vi "VCS Get Velocity Regulator Feed Forward.vi"(0 "axis in":cluster{"keyHandle":u32, "nodeId":u16}={"keyHandle"=0, "nodeId"=1}, 11 "error in (no error)":errorcluster) -> (4 "axis out":cluster{"keyHandle":u32, "nodeId":u16}={"keyHandle"=0, "nodeId"=1}, 6 "feed forward":T1, 15 "error out":errorcluster)   [LabVIEW 2010]
doc: "<B>VCS_GetVelocityRegulatorFeedForward</B> reads parameters for velocity regulation feed forward."
uses:
  Resources/EposCmd.dll
  Resources/EposCmd64.dll
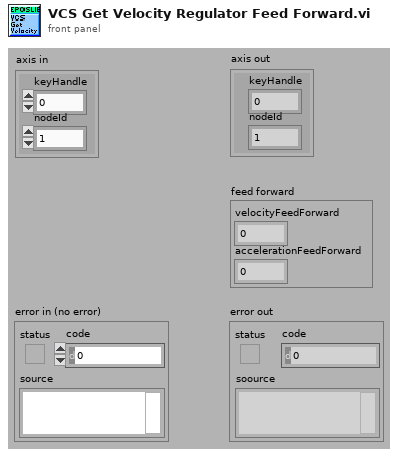
[diagram p1: front panel]
types:
  T1 = cluster{"velocityFeedForward":u16, "accelerationFeedForward":u16}
  T2 = cluster{"pVelocityFeedForward":u16, "pAccelerationFeedForward":u16}
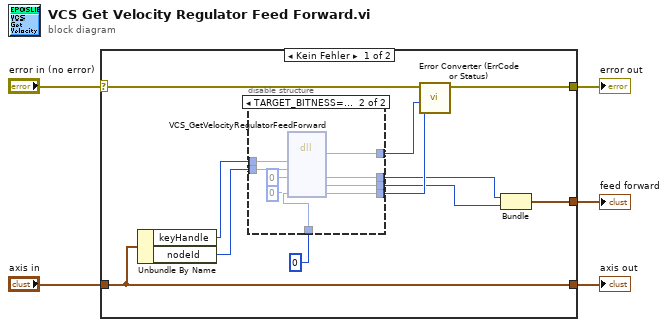
[diagram p0: block diagram]
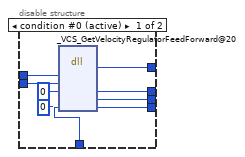
[diagram p2: hidden frame]
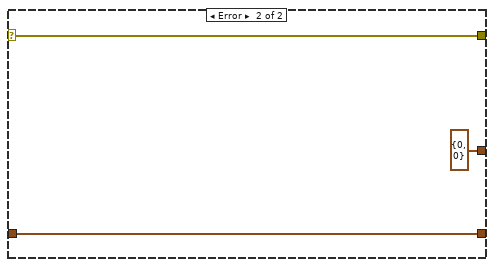
[diagram p3: hidden frame]
diagram:
  n1 = case shown="Kein Fehler" "error in (no error)" {
    selector: "error in (no error)" -> [w14 w36]
    tunnel: "axis in" -> [w16 w37]
    tunnel: [w16 w37] -> w4
    tunnel: [w15 w36] -> w3
    tunnel: [w6 T2 {"pVelocityFeedForward"=0, "pAccelerationFeedForward"=0}] -> w1
    frame No Error {
      n2 = Unbundle By Name(w16) -> ("keyHandle"=w12:u32, "nodeId"=w11:u16)
      n3 = disable-structure shown="TARGET_BITNESS==64" {
        disable-tunnel: u32 0 ("pErrorCode") -> [w25 w34]
        disable-tunnel: w12 -> [w24 w33]
        disable-tunnel: w11 -> [w23 w32]
        disable-tunnel: [w20 w29] -> w10
        disable-tunnel: [w19 w28] -> w9
        disable-tunnel: [w18 w27] -> w8
        disable-tunnel: [w17 w26] -> w7
        frame condition #0 (active) {
          n4 = dll-call lib="C:/Temp/maxon EPOS/Resources/EposCmd.*" fn="_VCS_GetVelocityRegulatorFeedForward@20" ("EposCmd.dll:_VCS_GetPositionRegulatorFeedForward@20")("KeyHandle"=w24, "NodeId"=w23, "pVelocityFeedForward"=u16 0, "pAccelerationFeedForward"=u16 0, "pErrorCode"=w25) -> (w19:i32, "pVelocityFeedForward"=w18:u16, "pAccelerationFeedForward"=w17:u16, "pErrorCode"=w20:u32)  [unwired: 5 in, 2 out]
        }
        frame condition #1 {
          n5 = dll-call lib="C:/setup/Resources/EposCmd64.*" fn="VCS_GetVelocityRegulatorFeedForward" ("EposCmd.dll:_VCS_GetPositionRegulatorFeedForward@20")("KeyHandle"=w33, "NodeId"=w32, "pVelocityFeedForward"=u16 0, "pAccelerationFeedForward"=u16 0, "pErrorCode"=w34) -> ("Rückgabetyp"=w28:i32, "pVelocityFeedForward"=w27:u16, "pAccelerationFeedForward"=w26:u16, "pErrorCode"=w29:u32)  [unwired: 5 in, 2 out]
        }
      }
      n6 = call "Error Converter (ErrCode or Status).vi"("error code"=w10, "return type"=w9, "error in (no error)"=w14) -> ("error out"=w15:errorcluster)  [unwired: 7 in]
      n7 = Bundle("pVelocityFeedForward"=w8, "pAccelerationFeedForward"=w7) -> (w6:T2)  [unwired: 1 in]
    }
    frame Error {
    }
  }
  "error out" <- w3
  "axis out" <- w4
  "feed forward" <- w1
